vi "Omni-teste-1.vi"() -> ()   [LabVIEW 2012]
panel:
  in  "stop":bool
  in  "Integration Time":i32
  out "Number of Spectrometers":i32
  out "XY Graph":T1(graph)
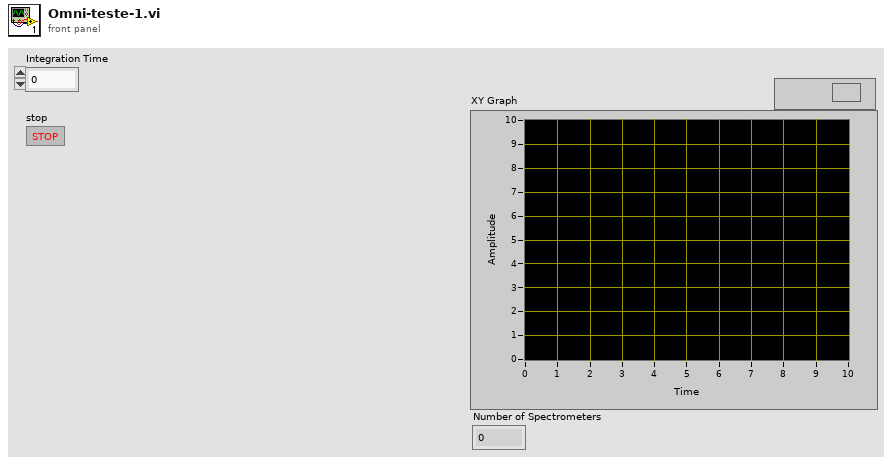
[diagram p1: front panel]
types:
  T1 = cluster{"WL Values":dbl[], "Spectrum Values":dbl[]}
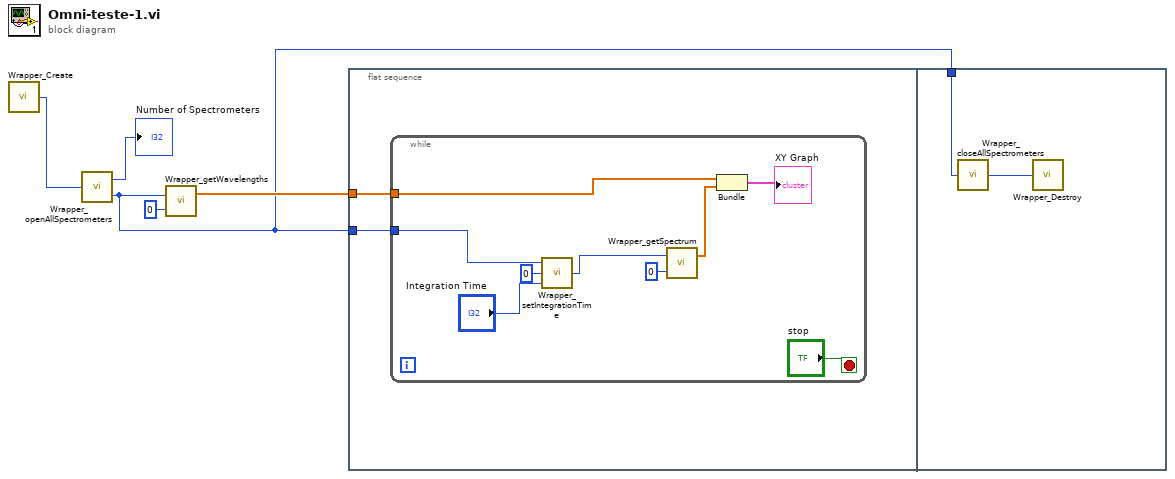
[diagram p0: block diagram]
diagram:
  n1 = call "Wrapper_Create.vi"() -> ("Wrapper"=w5:u32)
  n2 = call "Wrapper_openAllSpectrometers.vi"("Wrapper In"=w5) -> ("Number of Spectrometers"=→"Number of Spectrometers":i32, "Wrapper Out"=w1:u32)
  n3 = call "Wrapper_getWavelengths.vi"("Index"=0, "Wrapper"=w1) -> ("WL Values"=w2:dbl[])  [unwired: 1 out]
  n4 = flat-sequence {
    tunnel: w2 -> [w7]
    tunnel: w1 -> [w6]
    tunnel: w1 -> [w18]
    frame #0 {
      n5 = while {
        tunnel: w7 -> [w16]
        tunnel: w6 -> [w9]
        stop <- "stop" stop-if-true
        n6 = call "Wrapper_setIntegrationTime.vi"("Integration Time"="Integration Time", "Index"=0, "Wrapper In"=w9) -> ("Wrapper Out"=w12:u32)
        n7 = call "Wrapper_getSpectrum.vi"("Index"=0, "Wrapper"=w12) -> ("Spectrum Values"=w15:dbl[])  [unwired: 1 out]
        n8 = Bundle("WL Values"=w16, "Spectrum Values"=w15) -> (→"XY Graph":T1)  [unwired: 1 in]
      }
    }
    frame #1 {
      n9 = call "Wrapper_closeAllSpectrometers.vi"("Wrapper In"=w18) -> ("Wrapper Out"=w17:u32)
      n10 = call "Wrapper_Destroy.vi"("Wrapper"=w17) -> ()
    }
  }
